vi "DRAM FIFO test.vi"() -> ()   [LabVIEW 2019]
uses:
  <instrlib>/FlexRIO/DRAM FIFO/v2/FPGA/DRAM FIFO/DRAM FIFO Status.ctl
  <instrlib>/FlexRIO/DRAM FIFO/v2/FPGA/DRAM FIFO/FIFO Depth.ctl
  <vilib>/Platform/TimedLoop/XDataNode/timing_clust.ctl
  <vilib>/Platform/TimedLoop/XDataNode/nitl_modes.ctl
  <vilib>/Platform/TimedLoop/XDataNode/wakeup.ctl
  <instrlib>/FlexRIO/DRAM FIFO/v2/FPGA/DRAM FIFO/dynamic arbitration select.ctl
  <instrlib>/FlexRIO/DRAM FIFO/v2/FPGA/DRAM FIFO/Private/DRAM FIFO U512/Create 512x1 DRAM FIFO.vi
  <vilib>/rvi/Emulation/niFpgaSctlEmulationGetInTimedLoop.vi
  <vilib>/rvi/Emulation/niFpgaEmulationReportErrorSimple.vi
  <vilib>/rvi/Emulation/niFpgaGetClockAttributes.vi
  <vilib>/rvi/Emulation/niFpgaCriticalErrorInLSC.vi
  <vilib>/rvi/interface/RandomDataEmulation/nirviRandomDataMultiElementFPGAFIFO.vi
  <instcachedir>/0/nirviRandomDataMultiElementFPGAFIFO_1ED88BA00AC641F388A9B1FAA20E354D.lvgen/nirviRandomDataMultiElementFPGAFIFO_1ED88BA00AC641F388A9B1FAA20E354D_003.vi
  <vilib>/rvi/interface/RandomDataEmulation/niFpgaRandomDataHandleErrors.vi
  <instrlib>/_niInstr/Data Formatting/v1/FPGA/Private/Convert/FXP(+-,12,1) array to Boolean Array.vi
  <instrlib>/FlexRIO/DRAM FIFO/v2/FPGA/DRAM FIFO/Unpack Boolean Array.vi
  <instrlib>/_niInstr/Data Formatting/v1/FPGA/Private/Convert/Boolean Array to FXP(+-,12,1) Array.vi
  <instrlib>/FlexRIO/DRAM FIFO/v2/FPGA/DRAM FIFO/Pack Boolean Array.vi
  <vilib>/Platform/TimedLoop/XDataNode/XDataNode.xnode
  <vilib>/rvi/DataTransferAndStorage/Container/XNode/niFpgaContainer.xnode
  <vilib>/rvi/interface/RandomDataEmulation/nirviRandomDataFpgaMultiElementTemplate.vi
  <instrlib>/FlexRIO/DRAM FIFO/v2/FPGA/DRAM FIFO/DRAM FIFO v2 FPGA.lvclass
  <vilib>/Platform/TimedLoop/XDataNode/XDNodeRunTimeDep.lvlib
  <instrlib>/_niInstr/Data Formatting/v1/FPGA/niInstr Data Formatting v1 FPGA.lvlib
  <instrlib>/FlexRIO/DRAM FIFO/v2/FPGA/DRAM FIFO/Private/DRAM FIFO U512/DRAM FIFO U512 v2 FPGA.lvclass
panel:
  out "DRAM highwater":u32
  out "reset in progress?":bool
  in  "reset DRAM":bool
  in  "enable stream":bool
  out "status":T1
  in  "reset":bool
  out "elements per valid output":i32
  in  "dram.flush":bool
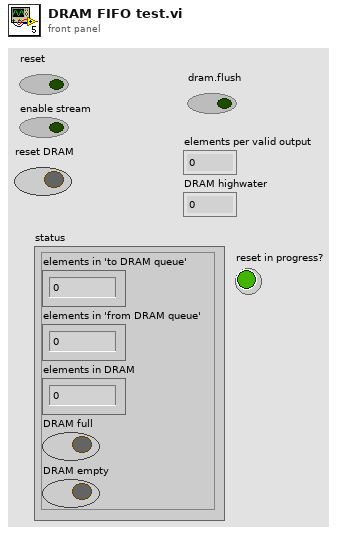
[diagram p1: front panel]
types:
  T1 = typedef "DRAM FIFO v2 FPGA.lvclass/DRAM FIFO Status.ctl" = cluster{"elements in 'to DRAM queue'":u32, "elements in 'from DRAM queue'":u32, "elements in DRAM":u32, "DRAM full":bool, "DRAM empty":bool}
  T2 = typedef "DRAM FIFO v2 FPGA.lvclass/FIFO Depth.ctl" = u8
  T3 = typedef "XDNodeRunTimeDep.lvlib/timing_clust.ctl" = cluster{"Expected End [f-1]":u64, "Actual End [f-1]":u64, "Finished Late? [f-1]":bool, "Expected End [i-1]":u64, "Actual End [i-1]":u64, "Finished Late? [i-1]":bool, "Expected Start [i]":u64, "Actual Start [i]":u64, "Expected Start [f]":u64, "Actual Start [f]":u64, "Source Name":string, "Structure Name":string, "Period":i64, "Deadline":i64, "Offset":i64, "Start":i64, "Priority":i32, "Timeout":i32, "Mode":T4, "Wakeup Reason":T5, "Error":errorcluster, "Source Type":string, "Secondary Source Type":string, "Global End Time":u64, "Global Start Time":u64, "Frame Duration":u64, "Iteration Duration":u64, "Assigned CPU":i32, "I/O Scan Engine Mode":u32}
  T4 = typedef "XDNodeRunTimeDep.lvlib/nitl_modes.ctl" = enum32{"No Change", "Process missed periods, maintain original phase", "Discard missed periods, maintain original phase", "Process missed periods, ignore original phase", "Discard missed periods, ignore original phase"}
  T5 = typedef "XDNodeRunTimeDep.lvlib/wakeup.ctl" = enum32{"Normal", "Aborted", "Asynchronous wakeup", "Timing source error", "Timed loop error", "Timeout"}
  T6 = typedef "DRAM FIFO v2 FPGA.lvclass/dynamic arbitration select.ctl" = enum16{"none", "dynamic (priority writes)", "dynamic (priority reads)"}
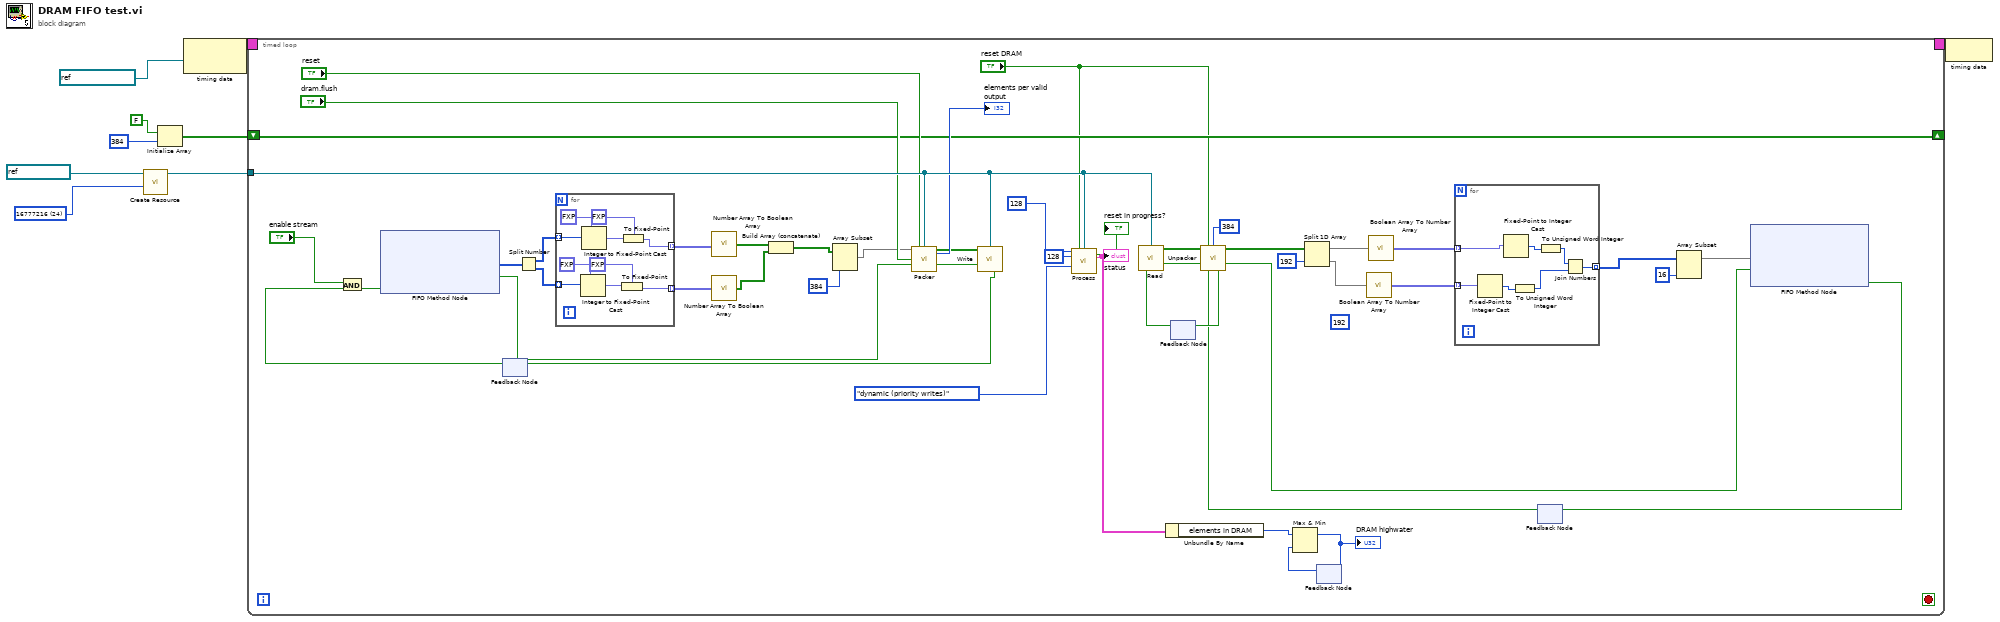
[diagram p0: block diagram]
diagram:
  w6 = T2 24 items=["4"=2, "8"=3, "16"=4, "32"=5, "64"=6, "128"=7, "256"=8, "512"=9, "1024"=10, "2048"=11, "4096"=12, "8192"=13, "16384"=14, "32768"=15, "65536"=16, "131072"=17, "262144"=18, "524288"=19, "1048576"=20, "2097152"=21, "4194304"=22, "8388608"=23, "16777216"=24, "33554432"=25, "67108864"=26, "134217728"=27, "268435456"=28, "536870912"=29, "1073741824"=30, "2147483648"=31, "4294967296"=32] ("actual # of DRAM elements")
  n1 = call-poly <instrlib>:"Create Resource.vi"("actual # of DRAM elements"=w6, "memory refnum"=refnum<k21> "RX memo") -> ("DRAM FIFO ref out"=w5:refnum<class "DRAM FIFO v2 FPGA.lvclass">)  [unwired: 9 in]
  n2 = Initialize Array(FALSE, 384 ("length")) -> (w1:bool[])
  n3 = node-c288(refnum<k21> "DRAM Clock" ("Source Name")) -> (w9:T3)
  n4 = timed-loop {
    timing: w9 -> [_]
    timing-out: [_] -> w8
    tunnel: w5 -> [w55]
    shift-right: [w36] -> _
    shift-left: w1 -> [w36]
    stop <- _ stop-if-true
    (unwired) 192 ("index")
    n5 = feedback #1() -> (w40:bool)  [unwired: 1 in]
    n6 = And(x="enable stream", y=w40) -> (x .and. y?=w39:bool)
    n7 = xnode ("FIFO Method Node")("Ready for Output"=w39) -> ("Element"=w32:u32[], "Output Valid"=w37:bool)  [unwired: 1 in, 1 out]
    n8 = Split Number(x=w32) -> (hi(x)=w31:u16[], lo(x)=w30:u16[])
    n9 = for {
      tunnel: w31 -> [w74] mode=indexing
      tunnel: w30 -> [w67] mode=indexing
      tunnel: [w66] -> w29 mode=indexing
      tunnel: [w65] -> w24 mode=indexing
      n10 = Integer to Fixed-Point Cast(fixed-point type=fxp<+/-,16,1> 0.0, integer=w67) -> (fixed-point=w69:fxp<+/-,16,1>)
      n11 = Integer to Fixed-Point Cast(fixed-point type=fxp<+/-,16,1> 0.0, integer=w74) -> (fixed-point=w72:fxp<+/-,16,1>)
      n12 = To Fixed-Point(fixed-point type=fxp<+/-,12,1> 0.0, number=w69) -> (fixed-point=w65:fxp<+/-,12,1>)
      n13 = To Fixed-Point(fixed-point type=fxp<+/-,12,1> 0.0, number=w72) -> (fixed-point=w66:fxp<+/-,12,1>)
    }
    n14 = call-poly <instrlib>:"Number Array To Boolean Array.vi"("data in"=w29) -> ("data out"=w28:bool[])  [unwired: 14 in]
    n15 = call-poly <instrlib>:"Number Array To Boolean Array.vi"("data in"=w24) -> ("data out"=w23:bool[])  [unwired: 14 in]
    n16 = Build Array (concatenate)(w28, w23) -> (w25:bool[])
    n17 = Array Subset(array=w25, length=384) -> (w26:bool[])  [unwired: 1 in]
    n18 = call-poly <instrlib>:"Packer.vi"("data in"=w26, "reset"="reset", "DRAM FIFO in"=w55, "flush data"="dram.flush", "input valid"=w37) -> ("elements per valid output"=→"elements per valid output":i32, "data out"=w47:bool[], "output valid"=w48:bool)  [unwired: 8 in]
    n19 = call <instrlib>:"Write.vi"("element"=w47, "DRAM FIFO ref in"=w55, "input valid"=w48) -> ("ready for input"=w41:bool)  [unwired: 12 in]
    n20 = feedback-in #1(w41) -> ()
    n21 = call <instrlib>:"Process.vi"("write grant time (clock ticks)"=u16 128, "reset DRAM"="reset DRAM", "DRAM FIFO ref in"=w55, "read grant time (clock ticks)"=u16 128, "dynamic arbitration"=dynamic_arbitration_select."dynamic (priority writes)") -> ("reset in progress?"=→"reset in progress?":bool, "status"=w13:T1)  [unwired: 9 in]
    "status" <- w13
    n22 = Unbundle By Name(w13) -> ("elements in DRAM"=w12:u32)
    n23 = feedback #2() -> (w51:bool)  [unwired: 1 in]
    n24 = call <instrlib>:"Read.vi"("DRAM FIFO ref in"=w55, "ready for output"=w51) -> ("element"=w54:bool[], "output valid"=w53:bool)  [unwired: 12 in]
    n25 = feedback #3() -> (w10:u32)  [unwired: 1 in]
    n26 = Max & Min(x=w12, y=w10) -> (max(x,y)=w11:u32)  [unwired: 1 out]
    "DRAM highwater" <- w11
    n27 = feedback-in #3(w11) -> ()
    n28 = feedback #4() -> (w44:bool)  [unwired: 1 in]
    n29 = call-poly <instrlib>:"Unpacker.vi"("packed data in"=w54, "reset"="reset DRAM", "output data size (bits)"=u16 384, "input valid"=w53, "ready for output"=w44) -> ("unpacked data out"=w21:bool[], "output valid"=w43:bool, "ready for input"=w52:bool)  [unwired: 8 in]
    n30 = feedback-in #2(w52) -> ()
    n31 = Split 1D Array(array=w21, index=192) -> (first subarray=w19:bool[], second subarray=w18:bool[])
    n32 = call-poly <instrlib>:"Boolean Array To Number Array.vi"("data in"=w18) -> ("data out"=w17:fxp<+/-,12,1>[])  [unwired: 14 in]
    n33 = call-poly <instrlib>:"Boolean Array To Number Array.vi"("data in"=w19) -> ("data out"=w22:fxp<+/-,12,1>[])  [unwired: 14 in]
    n34 = for {
      tunnel: w22 -> [w62] mode=indexing
      tunnel: w17 -> [w60] mode=indexing
      tunnel: [w64] -> w14 mode=indexing
      n35 = Fixed-Point to Integer Cast(1:w60) -> (0:w61:i16)
      n36 = Fixed-Point to Integer Cast(1:w62) -> (0:w63:i16)
      n37 = To Unsigned Word Integer(number=w61) -> (unsigned 16bit integer=w59:u16)
      n38 = To Unsigned Word Integer(number=w63) -> (unsigned 16bit integer=w58:u16)
      n39 = Join Numbers(hi=w58, lo=w59) -> ((hi.lo)=w64:u32)
    }
    n40 = Array Subset(array=w14, length=16) -> (w16:u32[])  [unwired: 1 in]
    n41 = xnode ("FIFO Method Node")("Element"=w16, "Input Valid"=w43) -> ("Ready for Input"=w45:bool)  [unwired: 1 in, 1 out]
    n42 = feedback-in #4(w45) -> ()
  }
  n43 = node-c288(w8) -> ()
